vi "Command Transfer Group.vi"(8 "error in (no error)":errorcluster, 9 "Command":T1=enum."Rx", 10 "Transfer Group":refnum<class "Transfer Group.lvclass">, 11 "Plugin Interface in":refnum<class "Plugin Interface.lvclass">) -> (0 "error out":errorcluster, 3 "Plugin Interface out":refnum<class "Plugin Interface.lvclass">)   [LabVIEW 2017, in "DSF Core.lvlib" / "Plugin Interface.lvclass"]
uses:
  Plugin Interface.lvclass
  C:/Git/DSF/Data Sharing Framework/Source/Core/Engine/Classes/Interfaces/Interface/Interface.lvclass
  Transfer Group/Transfer Group.lvclass
  Command.ctl
  Transfer Group/Transfer Group.lvclass/Transfer Group.ctl
  Timing/Timing.lvclass/Timing.ctl
  Command Data.ctl
  Command Parameters.ctl
  Interface/Interface.lvclass/Interface.ctl
  Debug/FIFO Flags/FIFO Flags.lvclass/FIFO Flags.ctl
  Write Plugin Command.vi
  Interface/Write Command.vi
  Interface/Get Command FIFO.vi
  Interface/Write RT FIFO(16B).vi
  Interface/Get Debug Flags.vi
  Debug/FIFO Flags/Get Infinite Timeouts.vi
  Interface/Errors.vi
  Interface/Command Timeout.vi
  Timing/Timing.lvclass
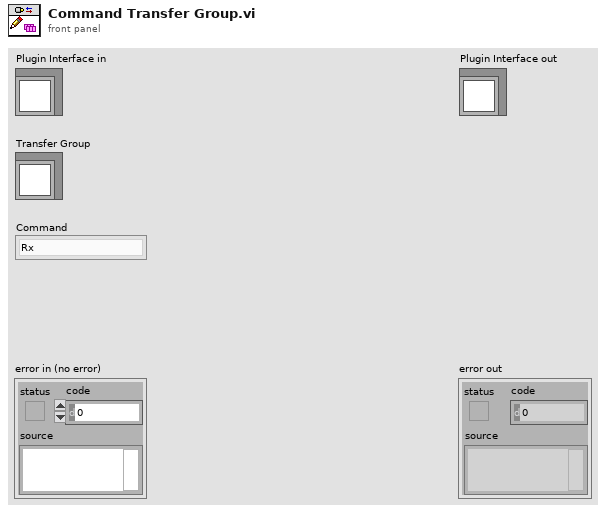
[diagram p1: front panel]
types:
  T1 = typedef "DSF Core.lvlib/Plugin Interface.lvclass/Command.ctl" = enum8{"Set Base Pointer", "Rx", "Tx", "Shutdown"}
  T2 = cluster{"Transfer Group ID":i32, "unused":i32, "Transfer Group iteration":u64}
  T3 = typedef "DSF Core.lvlib/Plugin Interface.lvclass/Command Parameters.ctl" = cluster{"arg1":u64, "arg2":u64}
  T4 = typedef "DSF Core.lvlib/Plugin Interface.lvclass/Command Data.ctl" = cluster{"Command":T1, "Command Parameters":T3}
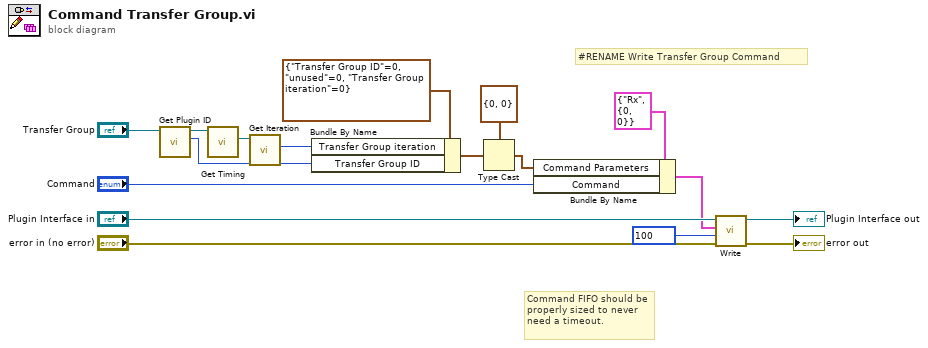
[diagram p0: block diagram]
diagram:
  # "#RENAME Write Transfer Group Command"
  # "Command FIFO should be properly sized to never need a timeout."
  n1 = call "Get Plugin ID.vi"("Transfer Group in"="Transfer Group") -> ("plugin id"=w10:i32, "Transfer Group out"=w9:refnum<class "Transfer Group.lvclass">)  [unwired: 9 in]
  n2 = call "Get Timing.vi"("Transfer Group in"=w9) -> ("Timing"=w8:refnum<class "Timing.lvclass">)  [unwired: 9 in, 1 out]
  n3 = call "Get Iteration.vi"("Timing in"=w8) -> ("Iteration"=w7:u64)  [unwired: 9 in, 1 out]
  n4 = Bundle By Name(cluster=T2 {"Transfer Group ID"=0, "unused"=0, "Transfer Group iteration"=0}, "Transfer Group iteration"=w7, "Transfer Group ID"=w10) -> (w11:T2)
  n5 = Type Cast(type=T3 {"arg1"=0, "arg2"=0} ("Command Parameters"), x=w11) -> (*(type *) &x=w13:T3)
  n6 = Bundle By Name(cluster=T4 {"Command"=enum."Rx", "Command Parameters"={"arg1"=0, "arg2"=0}} ("command"), "Command Parameters"=w13, "Command"="Command") -> (w1:T4)
  n7 = call-poly "Write.vi"("error in (no error)"="error in (no error)", "timeout in ms (0)"=100, "command"=w1, "Plugin Interface in"="Plugin Interface in") -> ("error out"=→"error out":errorcluster, "Plugin Interface out"=→"Plugin Interface out":refnum<class "Plugin Interface.lvclass">)  [unwired: 5 in, 1 out]
